vi "tools_openLibraryRootFolder.vi"   [LabVIEW 2023]
uses:
  TaskController/new.vi
  TaskController/TaskController.lvclass
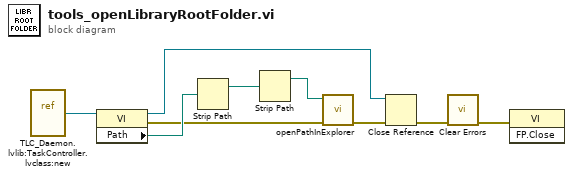
[diagram p0: block diagram]
diagram:
  n1 = vi-ref "TLC_Daemon.lvlib:TaskController.lvclass:new.vi"() -> (w9:refnum<vi>)
  n2 = property class="VI"(reference=w9) -> (reference out=w5:refnum<vi>, error out=w6:errorcluster, "Path"=w8:path)  [unwired: 1 in]
  n3 = Strip Path(path=w8) -> (stripped path=w7:path)  [unwired: 1 out]
  n4 = Strip Path(path=w7) -> (stripped path=w1:path)  [unwired: 1 out]
  n5 = call "openPathInExplorer.vi"("error in (no error)"=w6, "pathToOpen"=w1) -> ("error out"=w4:errorcluster)  [unwired: 9 in]
  n6 = Close Reference(reference=w5, error in (no error)=w4) -> (error out=w3:errorcluster)
  n7 = call <vilib>:"Clear Errors.vi"("error in (no error)"=w3) -> ("error out"=w2:errorcluster)  [unwired: 5 in, 1 out]
  n8 = invoke class="VI" method="FP.Close"(error in=w2) -> ()  [unwired: 2 in, 3 out]
